vi "Config OK Tab.vi"(8 "error in (no error)":errorcluster, 9 "String Selected":T1, 11 "Rigol DG822 Pulse in":refnum<class "Rigol DG822 Pulse.lvclass">) -> (0 "error out":errorcluster, 3 "Rigol DG822 Pulse out":refnum<class "Rigol DG822 Pulse.lvclass">)   [LabVIEW 2021, in "Rigol DG822 UI.lvlib" / "Rigol DG822 Pulse.lvlib" / "Rigol DG822 Pulse.lvclass"]
uses:
  Rigol DG822 Pulse.lvclass
  Rigol DG822 UI/lib/controls.llb/StringIndicatorSelected.ctl
  Rigol DG822 Pulse.lvclass/Rigol DG822 Pulse.ctl
  General/Files/lvlibp/Actors.lvlibp/Actors/Actors/Actors.lvclass
  D:/LabVIEW/General/Files/lvlibp/Actors.lvlibp/Actors/Actors/Actors.lvclass
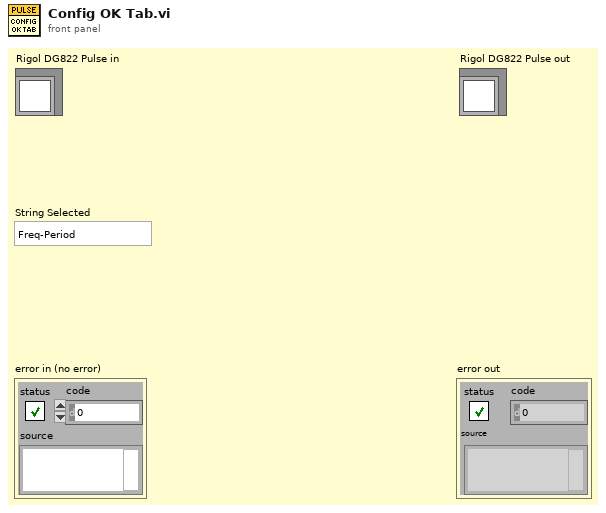
[diagram p1: front panel]
types:
  T1 = typedef "StringIndicatorSelected.ctl" = enum16{"Freq-Period", "Ampl-HighL", "Offset-LowL", "Phase", "Duty-Width", "RisEdge", "FallEdge"}
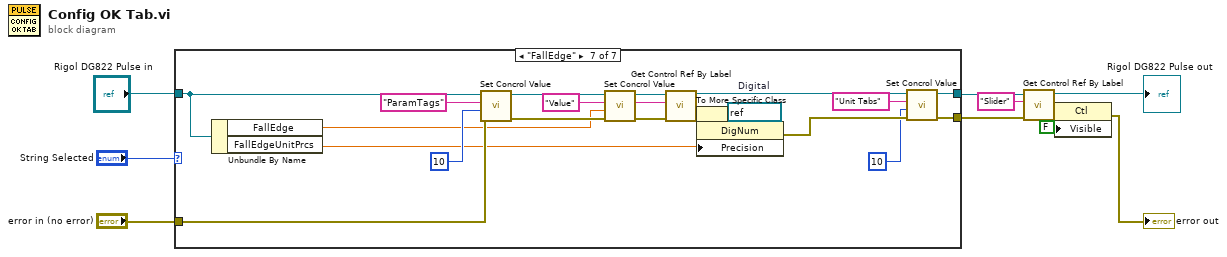
[diagram p0: block diagram]
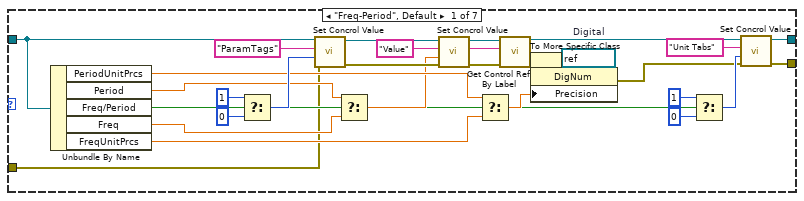
[diagram p2: hidden frame]
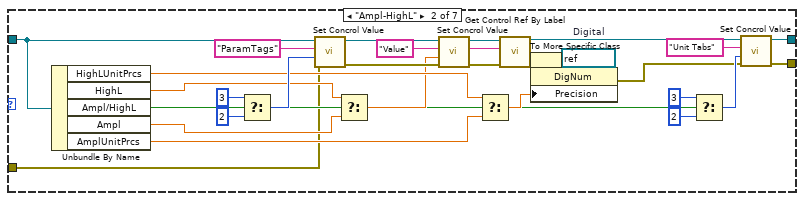
[diagram p3: hidden frame]
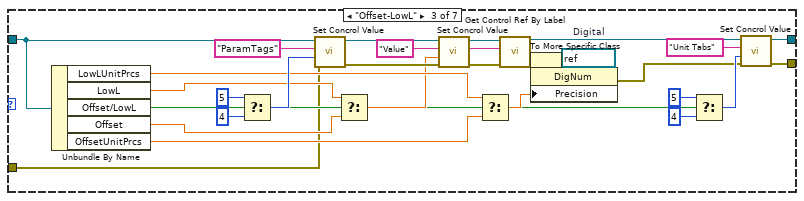
[diagram p4: hidden frame]
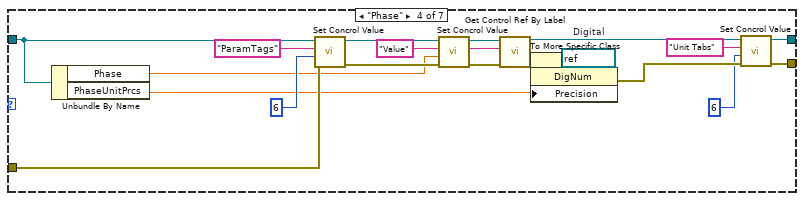
[diagram p5: hidden frame]
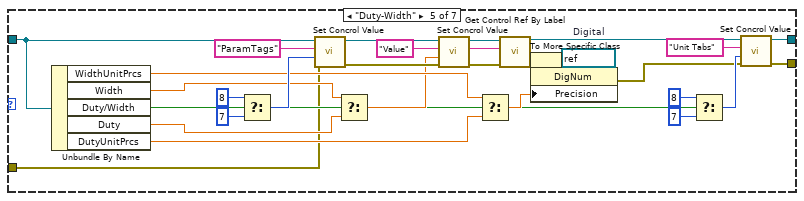
[diagram p6: hidden frame]
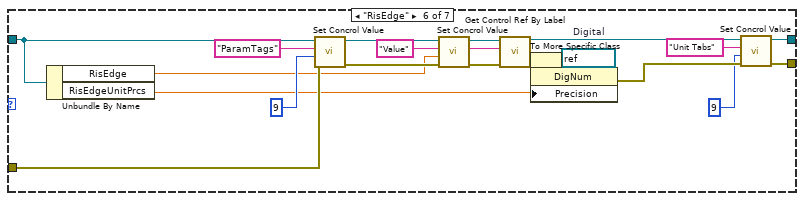
[diagram p7: hidden frame]
diagram:
  n1 = case shown="\"FallEdge\"" "String Selected" {
    tunnel: [w17 w47 w78 w112 w131 w165 w187] -> w3
    tunnel: "Rigol DG822 Pulse in" -> [w13 w60 w91 w119 w144 w172 w194]
    tunnel: [w14 w43 w74 w109 w127 w162 w184] -> w1
    tunnel: "error in (no error)" -> [w15 w44 w75 w110 w128 w163 w185]
    frame "Freq-Period", Default {
      w35 = refnum<vi> refnum  # Digital
      w26 = "Value" ("Control Label")
      n2 = Unbundle By Name(w13) -> ("PeriodUnitPrcs"=w20:dbl, "Period"=w23:dbl, "Freq/Period"=w16:bool, "Freq"=w22:dbl, "FreqUnitPrcs"=w21:dbl)
      n3 = Select(t=u16 1 ("ParamTags"), s=w16, f=u16 0 ("ParamTags")) -> (s? t:f=w27:u16)
      n4 = call "Set Concrol Value.vi"("error in (no error)"=w15, "Value"=w27, "Control Label"="ParamTags", "Actors in"=w13) -> ("error out"=w25:errorcluster, "Actors out"=w29:refnum<class "Rigol DG822 Pulse.lvclass">)  [unwired: 6 in]
      n5 = Select(t=w23, s=w16, f=w22) -> (s? t:f=w19:dbl)
      n6 = call "Set Concrol Value.vi"("error in (no error)"=w25, "Value"=w19, "Control Label"=w26, "Actors in"=w29) -> ("error out"=w24:errorcluster, "Actors out"=w28:refnum<class "Rigol DG822 Pulse.lvclass">)  [unwired: 6 in]
      n7 = Select(t=w20, s=w16, f=w21) -> (s? t:f=w36:dbl)
      n8 = call "Get Control Ref By Label.vi"("error in (no error)"=w24, "Control Label"=w26, "Actors in"=w28) -> ("error out"=w37:errorcluster, "Control Ref"=w33:refnum<vi>, "Actors out"=w18:refnum<class "Rigol DG822 Pulse.lvclass">)  [unwired: 6 in]
      n9 = To More Specific Class(target class=w35, reference=w33, error in=w37) -> (specific class reference=w34:refnum<vi>, error out=w38:errorcluster)
      n10 = property class="DigNum"(reference=w34, error in=w38, "Precision"=w36) -> (error out=w12:errorcluster)  [unwired: 1 out]
      n11 = Select(t=u16 1 ("ParamTags"), s=w16, f=u16 0 ("ParamTags")) -> (s? t:f=w42:u16)
      n12 = call "Set Concrol Value.vi"("error in (no error)"=w12, "Value"=w42, "Control Label"="Unit Tabs", "Actors in"=w18) -> ("error out"=w14:errorcluster, "Actors out"=w17:refnum<class "Rigol DG822 Pulse.lvclass">)  [unwired: 6 in]
    }
    frame "Ampl-HighL" {
      w66 = refnum<vi> refnum  # Digital
      w56 = "Value" ("Control Label")
      n13 = Unbundle By Name(w60) -> ("HighLUnitPrcs"=w50:dbl, "HighL"=w53:dbl, "Ampl/HighL"=w45:bool, "Ampl"=w52:dbl, "AmplUnitPrcs"=w51:dbl)
      n14 = Select(t=u16 3 ("ParamTags"), s=w45, f=u16 2 ("ParamTags")) -> (s? t:f=w57:u16)
      n15 = call "Set Concrol Value.vi"("error in (no error)"=w44, "Value"=w57, "Control Label"="ParamTags", "Actors in"=w60) -> ("error out"=w55:errorcluster, "Actors out"=w59:refnum<class "Rigol DG822 Pulse.lvclass">)  [unwired: 6 in]
      n16 = Select(t=w53, s=w45, f=w52) -> (s? t:f=w49:dbl)
      n17 = call "Set Concrol Value.vi"("error in (no error)"=w55, "Value"=w49, "Control Label"=w56, "Actors in"=w59) -> ("error out"=w54:errorcluster, "Actors out"=w58:refnum<class "Rigol DG822 Pulse.lvclass">)  [unwired: 6 in]
      n18 = Select(t=w50, s=w45, f=w51) -> (s? t:f=w67:dbl)
      n19 = call "Get Control Ref By Label.vi"("error in (no error)"=w54, "Control Label"=w56, "Actors in"=w58) -> ("error out"=w68:errorcluster, "Control Ref"=w64:refnum<vi>, "Actors out"=w48:refnum<class "Rigol DG822 Pulse.lvclass">)  [unwired: 6 in]
      n20 = To More Specific Class(target class=w66, reference=w64, error in=w68) -> (specific class reference=w65:refnum<vi>, error out=w69:errorcluster)
      n21 = property class="DigNum"(reference=w65, error in=w69, "Precision"=w67) -> (error out=w46:errorcluster)  [unwired: 1 out]
      n22 = Select(t=u16 3 ("ParamTags"), s=w45, f=u16 2 ("ParamTags")) -> (s? t:f=w73:u16)
      n23 = call "Set Concrol Value.vi"("error in (no error)"=w46, "Value"=w73, "Control Label"="Unit Tabs", "Actors in"=w48) -> ("error out"=w43:errorcluster, "Actors out"=w47:refnum<class "Rigol DG822 Pulse.lvclass">)  [unwired: 6 in]
    }
    frame "Offset-LowL" {
      w97 = refnum<vi> refnum  # Digital
      w87 = "Value" ("Control Label")
      n24 = Unbundle By Name(w91) -> ("LowLUnitPrcs"=w81:dbl, "LowL"=w84:dbl, "Offset/LowL"=w76:bool, "Offset"=w83:dbl, "OffsetUnitPrcs"=w82:dbl)
      n25 = Select(t=u16 5 ("ParamTags"), s=w76, f=u16 4 ("ParamTags")) -> (s? t:f=w88:u16)
      n26 = call "Set Concrol Value.vi"("error in (no error)"=w75, "Value"=w88, "Control Label"="ParamTags", "Actors in"=w91) -> ("error out"=w86:errorcluster, "Actors out"=w90:refnum<class "Rigol DG822 Pulse.lvclass">)  [unwired: 6 in]
      n27 = Select(t=w84, s=w76, f=w83) -> (s? t:f=w80:dbl)
      n28 = call "Set Concrol Value.vi"("error in (no error)"=w86, "Value"=w80, "Control Label"=w87, "Actors in"=w90) -> ("error out"=w85:errorcluster, "Actors out"=w89:refnum<class "Rigol DG822 Pulse.lvclass">)  [unwired: 6 in]
      n29 = Select(t=w81, s=w76, f=w82) -> (s? t:f=w98:dbl)
      n30 = call "Get Control Ref By Label.vi"("error in (no error)"=w85, "Control Label"=w87, "Actors in"=w89) -> ("error out"=w99:errorcluster, "Control Ref"=w95:refnum<vi>, "Actors out"=w79:refnum<class "Rigol DG822 Pulse.lvclass">)  [unwired: 6 in]
      n31 = To More Specific Class(target class=w97, reference=w95, error in=w99) -> (specific class reference=w96:refnum<vi>, error out=w100:errorcluster)
      n32 = property class="DigNum"(reference=w96, error in=w100, "Precision"=w98) -> (error out=w77:errorcluster)  [unwired: 1 out]
      n33 = Select(t=u16 5 ("ParamTags"), s=w76, f=u16 4 ("ParamTags")) -> (s? t:f=w104:u16)
      n34 = call "Set Concrol Value.vi"("error in (no error)"=w77, "Value"=w104, "Control Label"="Unit Tabs", "Actors in"=w79) -> ("error out"=w74:errorcluster, "Actors out"=w78:refnum<class "Rigol DG822 Pulse.lvclass">)  [unwired: 6 in]
    }
    frame "Phase" {
      w123 = refnum<vi> refnum  # Digital
      w116 = "Value" ("Control Label")
      n35 = Unbundle By Name(w119) -> ("Phase"=w107:dbl, "PhaseUnitPrcs"=w106:dbl)
      n36 = call "Set Concrol Value.vi"("error in (no error)"=w110, "Value"=u16 6 ("ParamTags"), "Control Label"="ParamTags", "Actors in"=w119) -> ("error out"=w115:errorcluster, "Actors out"=w118:refnum<class "Rigol DG822 Pulse.lvclass">)  [unwired: 6 in]
      n37 = call "Set Concrol Value.vi"("error in (no error)"=w115, "Value"=w107, "Control Label"=w116, "Actors in"=w118) -> ("error out"=w114:errorcluster, "Actors out"=w117:refnum<class "Rigol DG822 Pulse.lvclass">)  [unwired: 6 in]
      n38 = call "Get Control Ref By Label.vi"("error in (no error)"=w114, "Control Label"=w116, "Actors in"=w117) -> ("error out"=w124:errorcluster, "Control Ref"=w121:refnum<vi>, "Actors out"=w113:refnum<class "Rigol DG822 Pulse.lvclass">)  [unwired: 6 in]
      n39 = To More Specific Class(target class=w123, reference=w121, error in=w124) -> (specific class reference=w122:refnum<vi>, error out=w125:errorcluster)
      n40 = property class="DigNum"(reference=w122, error in=w125, "Precision"=w106) -> (error out=w111:errorcluster)  [unwired: 1 out]
      n41 = call "Set Concrol Value.vi"("error in (no error)"=w111, "Value"=u16 6 ("ParamTags"), "Control Label"="Unit Tabs", "Actors in"=w113) -> ("error out"=w109:errorcluster, "Actors out"=w112:refnum<class "Rigol DG822 Pulse.lvclass">)  [unwired: 6 in]
    }
    frame "Duty-Width" {
      w150 = refnum<vi> refnum  # Digital
      w140 = "Value" ("Control Label")
      n42 = Unbundle By Name(w144) -> ("WidthUnitPrcs"=w134:dbl, "Width"=w137:dbl, "Duty/Width"=w129:bool, "Duty"=w136:dbl, "DutyUnitPrcs"=w135:dbl)
      n43 = Select(t=u16 8 ("ParamTags"), s=w129, f=u16 7 ("ParamTags")) -> (s? t:f=w141:u16)
      n44 = call "Set Concrol Value.vi"("error in (no error)"=w128, "Value"=w141, "Control Label"="ParamTags", "Actors in"=w144) -> ("error out"=w139:errorcluster, "Actors out"=w143:refnum<class "Rigol DG822 Pulse.lvclass">)  [unwired: 6 in]
      n45 = Select(t=w137, s=w129, f=w136) -> (s? t:f=w133:dbl)
      n46 = call "Set Concrol Value.vi"("error in (no error)"=w139, "Value"=w133, "Control Label"=w140, "Actors in"=w143) -> ("error out"=w138:errorcluster, "Actors out"=w142:refnum<class "Rigol DG822 Pulse.lvclass">)  [unwired: 6 in]
      n47 = Select(t=w134, s=w129, f=w135) -> (s? t:f=w151:dbl)
      n48 = call "Get Control Ref By Label.vi"("error in (no error)"=w138, "Control Label"=w140, "Actors in"=w142) -> ("error out"=w152:errorcluster, "Control Ref"=w148:refnum<vi>, "Actors out"=w132:refnum<class "Rigol DG822 Pulse.lvclass">)  [unwired: 6 in]
      n49 = To More Specific Class(target class=w150, reference=w148, error in=w152) -> (specific class reference=w149:refnum<vi>, error out=w153:errorcluster)
      n50 = property class="DigNum"(reference=w149, error in=w153, "Precision"=w151) -> (error out=w130:errorcluster)  [unwired: 1 out]
      n51 = Select(t=u16 8 ("ParamTags"), s=w129, f=u16 7 ("ParamTags")) -> (s? t:f=w157:u16)
      n52 = call "Set Concrol Value.vi"("error in (no error)"=w130, "Value"=w157, "Control Label"="Unit Tabs", "Actors in"=w132) -> ("error out"=w127:errorcluster, "Actors out"=w131:refnum<class "Rigol DG822 Pulse.lvclass">)  [unwired: 6 in]
    }
    frame "RisEdge" {
      w176 = refnum<vi> refnum  # Digital
      w169 = "Value" ("Control Label")
      n53 = Unbundle By Name(w172) -> ("RisEdge"=w160:dbl, "RisEdgeUnitPrcs"=w159:dbl)
      n54 = call "Set Concrol Value.vi"("error in (no error)"=w163, "Value"=u16 9 ("ParamTags"), "Control Label"="ParamTags", "Actors in"=w172) -> ("error out"=w168:errorcluster, "Actors out"=w171:refnum<class "Rigol DG822 Pulse.lvclass">)  [unwired: 6 in]
      n55 = call "Set Concrol Value.vi"("error in (no error)"=w168, "Value"=w160, "Control Label"=w169, "Actors in"=w171) -> ("error out"=w167:errorcluster, "Actors out"=w170:refnum<class "Rigol DG822 Pulse.lvclass">)  [unwired: 6 in]
      n56 = call "Get Control Ref By Label.vi"("error in (no error)"=w167, "Control Label"=w169, "Actors in"=w170) -> ("error out"=w177:errorcluster, "Control Ref"=w174:refnum<vi>, "Actors out"=w166:refnum<class "Rigol DG822 Pulse.lvclass">)  [unwired: 6 in]
      n57 = To More Specific Class(target class=w176, reference=w174, error in=w177) -> (specific class reference=w175:refnum<vi>, error out=w178:errorcluster)
      n58 = property class="DigNum"(reference=w175, error in=w178, "Precision"=w159) -> (error out=w164:errorcluster)  [unwired: 1 out]
      n59 = call "Set Concrol Value.vi"("error in (no error)"=w164, "Value"=u16 9 ("ParamTags"), "Control Label"="Unit Tabs", "Actors in"=w166) -> ("error out"=w162:errorcluster, "Actors out"=w165:refnum<class "Rigol DG822 Pulse.lvclass">)  [unwired: 6 in]
    }
    frame "FallEdge" {
      w198 = refnum<vi> refnum  # Digital
      w191 = "Value" ("Control Label")
      n60 = Unbundle By Name(w194) -> ("FallEdge"=w182:dbl, "FallEdgeUnitPrcs"=w181:dbl)
      n61 = call "Set Concrol Value.vi"("error in (no error)"=w185, "Value"=u16 10 ("ParamTags"), "Control Label"="ParamTags", "Actors in"=w194) -> ("error out"=w190:errorcluster, "Actors out"=w193:refnum<class "Rigol DG822 Pulse.lvclass">)  [unwired: 6 in]
      n62 = call "Set Concrol Value.vi"("error in (no error)"=w190, "Value"=w182, "Control Label"=w191, "Actors in"=w193) -> ("error out"=w189:errorcluster, "Actors out"=w192:refnum<class "Rigol DG822 Pulse.lvclass">)  [unwired: 6 in]
      n63 = call "Get Control Ref By Label.vi"("error in (no error)"=w189, "Control Label"=w191, "Actors in"=w192) -> ("error out"=w199:errorcluster, "Control Ref"=w196:refnum<vi>, "Actors out"=w188:refnum<class "Rigol DG822 Pulse.lvclass">)  [unwired: 6 in]
      n64 = To More Specific Class(target class=w198, reference=w196, error in=w199) -> (specific class reference=w197:refnum<vi>, error out=w200:errorcluster)
      n65 = property class="DigNum"(reference=w197, error in=w200, "Precision"=w181) -> (error out=w186:errorcluster)  [unwired: 1 out]
      n66 = call "Set Concrol Value.vi"("error in (no error)"=w186, "Value"=u16 10 ("ParamTags"), "Control Label"="Unit Tabs", "Actors in"=w188) -> ("error out"=w184:errorcluster, "Actors out"=w187:refnum<class "Rigol DG822 Pulse.lvclass">)  [unwired: 6 in]
    }
  }
  n67 = call "Get Control Ref By Label.vi"("error in (no error)"=w1, "Control Label"="Slider", "Actors in"=w3) -> ("error out"=w6:errorcluster, "Control Ref"=w5:refnum<vi>, "Actors out"=→"Rigol DG822 Pulse out":refnum<class "Rigol DG822 Pulse.lvclass">)  [unwired: 6 in]
  n68 = property class="Ctl"(reference=w5, error in=w6, "Visible"=FALSE) -> (error out=→"error out":errorcluster)  [unwired: 1 out]
